vi "read TBM configuration.vi"(8 "error in":errorcluster, 11 "Scan Engine editor node in":refnum<class "Scan Engine editor node.lvclass">) -> (0 "error out":errorcluster, 2 "configuration":refnum<class "TBM configuration.lvclass">, 3 "Scan Engine editor node out":refnum<class "Scan Engine editor node.lvclass">)   [LabVIEW 2013, in "Scan Engine editor node.lvclass"]
uses:
  Scan Engine editor node.lvclass
  <vilib>/NI/Tag Bus Module Framework/root configuration/TBM configuration.lvclass
  Scan Engine editor node.lvclass/Scan Engine editor node.ctl
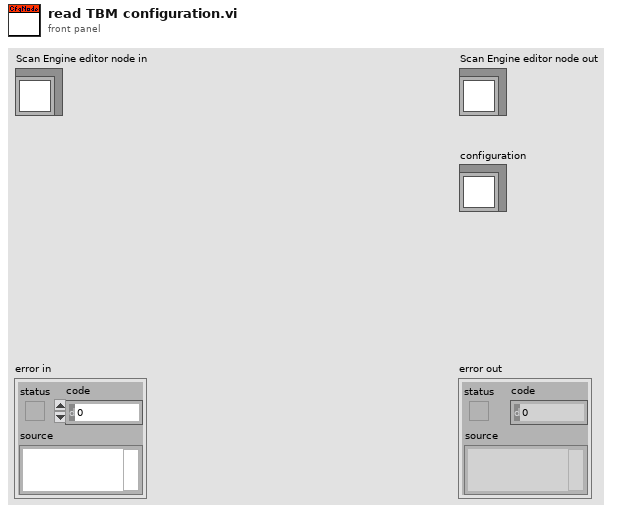
[diagram p1: front panel]
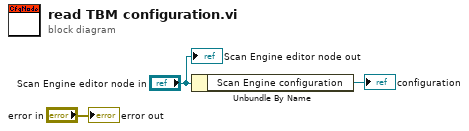
[diagram p0: block diagram]
diagram:
  n1 = Unbundle By Name("Scan Engine editor node in") -> ("Scan Engine configuration"=→"configuration":refnum<class "Scan Engine configuration.lvclass">)
  "error out" <- "error in"
  "Scan Engine editor node out" <- "Scan Engine editor node in"
